vi "ocr.vi"() -> ()   [LabVIEW 2011]
uses:
  <vilib>/vision/NI_Vision_Development_Module.lvlib
panel:
  in  "character set Path":path
  out "Path":path
  out "Image":T1(plugin-control)
  out "Read String:":string
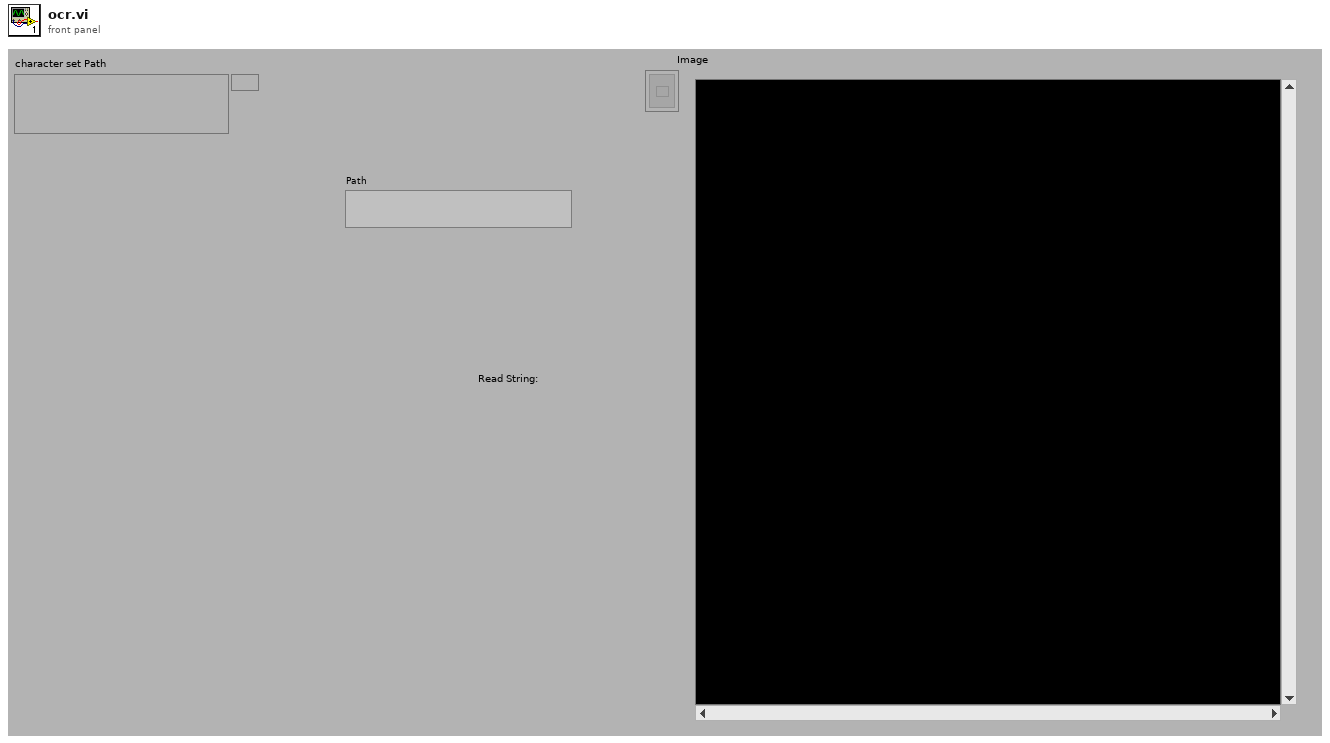
[diagram p1: front panel]
types:
  T1 = typedef "IMAQ Image.ctl" = refnum<image>
  T2 = cluster{"Global Rectangle":i32[], "Contours":cluster{"ID":enum32{"External", "Internal"}, "Type":u32, "Coordinates":i32[]}[]}
  T3 = enum32{"8 bits", "16 bits", "Float", "Complex", "RGB Chunky", "Compressed"}
  T4 = typedef "IMAQ OCR Session.ctl" = refnum<k1>
  T5 = cluster{"Global Rectangle":i32[], "Contours":cluster{"Contour Type":u32, "ROI Type":u32, "Points":i32[]}[]}
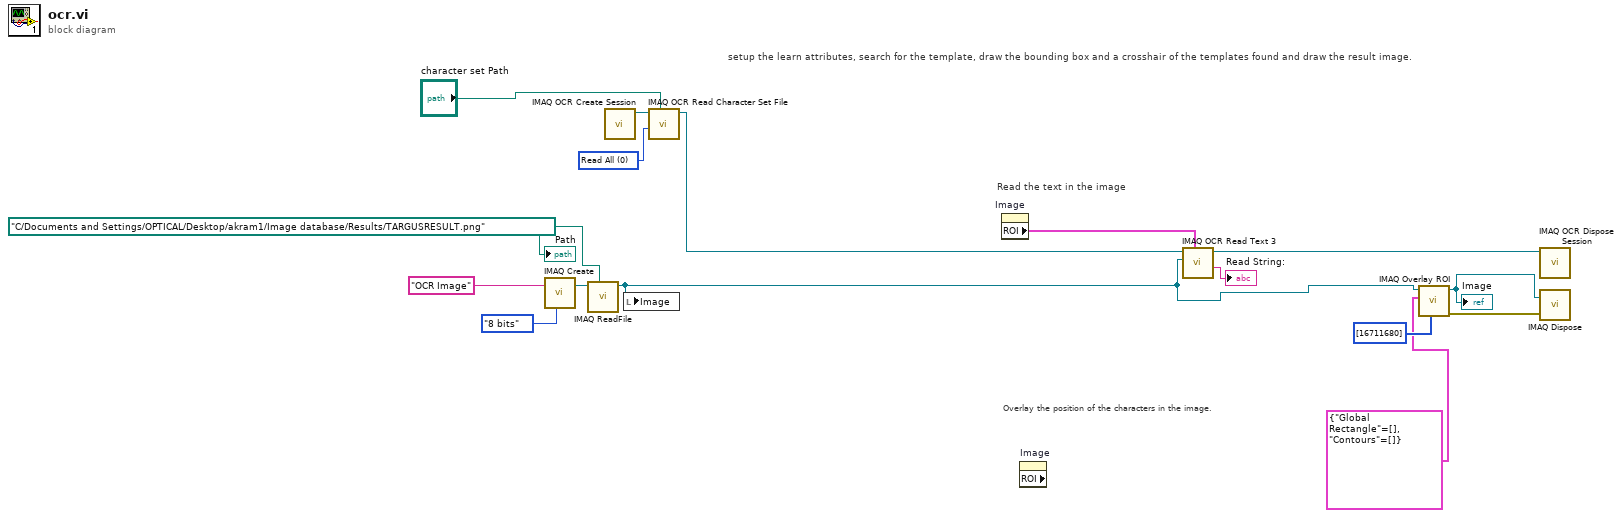
[diagram p0: block diagram]
diagram:
  w9 = 0 items=["Read All", "Read Character Set Only", "Read Properties Only"] ("Read Options")
  w11 = path "C:/Documents and Settings/OPTICAL/Desktop/akram1/Image database/Results/TARGUSRESULT.png" ("selected path")
  # "Read the text in the image"
  # "Overlay the position of the characters in the image."
  # "setup the learn attributes, search for the template, draw the bounding box and a crosshair of the templates found and draw the result image."
  n1 = call "IMAQ Create"("Image Name"="OCR Image", "Image Type"=T3."8 bits") -> ("New Image"=w10:T1)  [unwired: 2 in, 2 out]
  n2 = call "IMAQ ReadFile"("File Path"=w11, "Image"=w10) -> ("Image Out"=w4:T1)  [unwired: 3 in, 6 out]
  n3 = call "IMAQ OCR Create Session"() -> ("IMAQ OCR Session"=w8:T4)  [unwired: 1 in, 10 out]
  n4 = local write "Image"(w4) -> ()
  n5 = call "IMAQ OCR Read Character Set File"("File Path"="character set Path", "Read Options"=w9, "IMAQ OCR Session"=w8) -> ("IMAQ OCR Session (dup)"=w7:T4)  [unwired: 2 in, 6 out]
  n6 = property on="Image" class="ImageControl"() -> ("ROI"=w1:T5)  [unwired: 2 in, 2 out]
  n7 = property on="Image" class="ImageControl" props=["ROI"]() -> ()  [unwired: 2 in, 3 out]
  n8 = call "IMAQ OCR Read Text 3"("ROI Descriptor"=w1, "Image"=w4, "IMAQ OCR Session"=w7) -> ("Read String"=→"Read String:":string, "IMAQ OCR Session (dup)"=w14:T4)  [unwired: 2 in, 5 out]
  n9 = call "IMAQ Overlay ROI"("Colors (Green)"=u32[] [16711680], "ROI Descriptor"=T2 {"Global Rectangle"=[], "Contours"=[]} ("ROI Bounding Characters"), "Image"=w4) -> ("error out"=w12:errorcluster, "Image Out"=w13:T1)  [unwired: 3 in, 4 out]
  "Image" <- w13
  n10 = call "IMAQ OCR Dispose Session"("IMAQ OCR Session"=w14) -> ()  [unwired: 1 in, 10 out]
  n11 = call "IMAQ Dispose"("Image"=w13, "error in (no error)"=w12) -> ()  [unwired: 1 in, 4 out]
  "Path" <- w11
